vi "HackRF_Read_Int8.vi"(8 "error in (no error)":errorcluster, 10 "count":i32=1000, 11 "HackRF":T1) -> (0 "error out":errorcluster, 1 "Q data":i8[](array[numeric]), 2 "I data":i8[](array[numeric]), 3 "HackRF":T1)   [LabVIEW 2021]
uses:
  Users/fl1ckje/Downloads/LV_HackRF_FMreceiver-main/HackRF_Lib/HackRF_Ref.ctl
  C:/Users/fl1ckje/Downloads/LV_HackRF_FMreceiver-main/HackRF_Lib/NetHackrf.dll
  Users/fl1ckje/Downloads/LV_HackRF_FMreceiver-main/HackRF_Lib/NetHackrf.dll
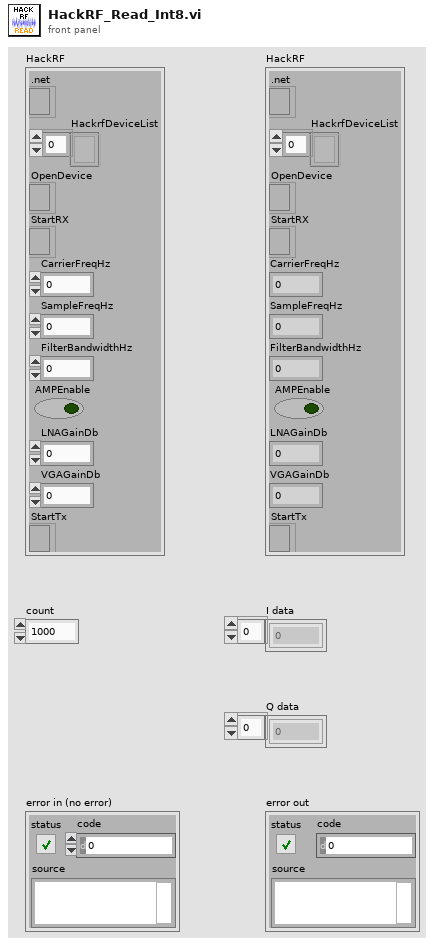
[diagram p1: front panel]
types:
  T1 = typedef "HackRF_Ref.ctl" = cluster{".net":refnum<k24>, "HackrfDeviceList":refnum<k24>[], "OpenDevice":refnum<k24>, "StartRX":refnum<k24>, "CarrierFreqHz":dbl, "SampleFreqHz":dbl, "FilterBandwidthHz":dbl, "AMPEnable":bool, "LNAGainDb":dbl, "VGAGainDb":dbl, "StartTx":refnum<k24>}
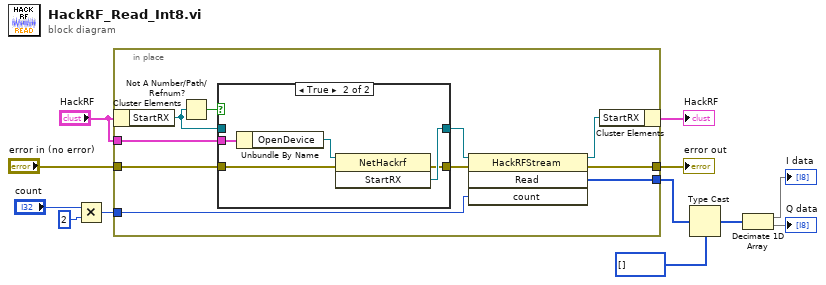
[diagram p0: block diagram]
diagram:
  n1 = Multiply(x="count", y=2) -> (x*y=w1:i32)
  n2 = in-place {
    in-place-border: "HackRF" -> [w21]
    in-place-border: w1 -> [w18]
    in-place-border: "error in (no error)" -> [w17]
    in-place-border: [w15] -> w10
    in-place-border: [w13] -> w8
    n3 = in-place-cluster #1("HackRF") -> ("StartRX"=w20:refnum<k24>)
    n4 = Not A Number/Path/Refnum?(number/path/refnum=w20) -> (NaN/Path/Refnum?=w22:bool)
    n5 = case shown="True" w22 {
      tunnel: [w24 w29] -> w19
      tunnel: w21 -> [_ w28]
      tunnel: w20 -> [w24 _]
      tunnel: w17 -> [w23 w25]
      tunnel: [w23 w26] -> w16
      frame False {
      }
      frame True {
        n6 = Unbundle By Name(w28) -> ("OpenDevice"=w27:refnum<k24>)
        n7 = invoke class="NetHackrf" method="StartRX"(reference=w27, error in=w25) -> (error out=w26:errorcluster, "StartRX"=w29:refnum<k24>)  [unwired: 1 in, 1 out]
      }
    }
    n8 = invoke class="HackRFStream" method="Read"(reference=w19, error in=w16, "count"=w18) -> (reference out=w14:refnum<k24>, error out=w15:errorcluster, "Read"=w13:u8[])  [unwired: 1 in, 1 out]
    n9 = in-place-cluster #1("StartRX"=w14) -> (→"HackRF":T1)
  }
  "error out" <- w10
  n10 = Type Cast(type=i8[] [] ("Read"), x=w8) -> (*(type *) &x=w6:i8[])
  n11 = Decimate 1D Array(w6) -> (→"I data":i8[], →"Q data":i8[])
